vi "数据时间对齐.vi"(9 "待对齐时间":T1 {"单位" items=["ug/L", "mg/L", "ppm", "mg/m3", "cm", "ppb", "ug/m3", "%", "nmol/mol", "umol/mol", "MPN/L", "MPN/100ml", "ng/m3", "NTU", "无量纲", "ms/cm", "us/cm", "℃", "mV", "万个/L"]}, 10 "对齐参考时间":T1 {"单位" items=["ug/L", "mg/L", "ppm", "mg/m3", "cm", "ppb", "ug/m3", "%", "nmol/mol", "umol/mol", "MPN/L", "MPN/100ml", "ng/m3", "NTU", "无量纲", "ms/cm", "us/cm", "℃", "mV", "万个/L"]}, 11 "已对齐时间输入":T1 {"单位" items=["ug/L", "mg/L", "ppm", "mg/m3", "cm", "ppb", "ug/m3", "%", "nmol/mol", "umol/mol", "MPN/L", "MPN/100ml", "ng/m3", "NTU", "无量纲", "ms/cm", "us/cm", "℃", "mV", "万个/L"]}) -> (3 "已对齐时间输出":T1 {"单位" items=["ug/L", "mg/L", "ppm", "mg/m3", "cm", "ppb", "ug/m3", "%", "nmol/mol", "umol/mol", "MPN/L", "MPN/100ml", "ng/m3", "NTU", "无量纲", "ms/cm", "us/cm", "℃", "mV", "万个/L"]})   [LabVIEW 2022 SP3, in "斯坦道总磷总氮.lvlib"]
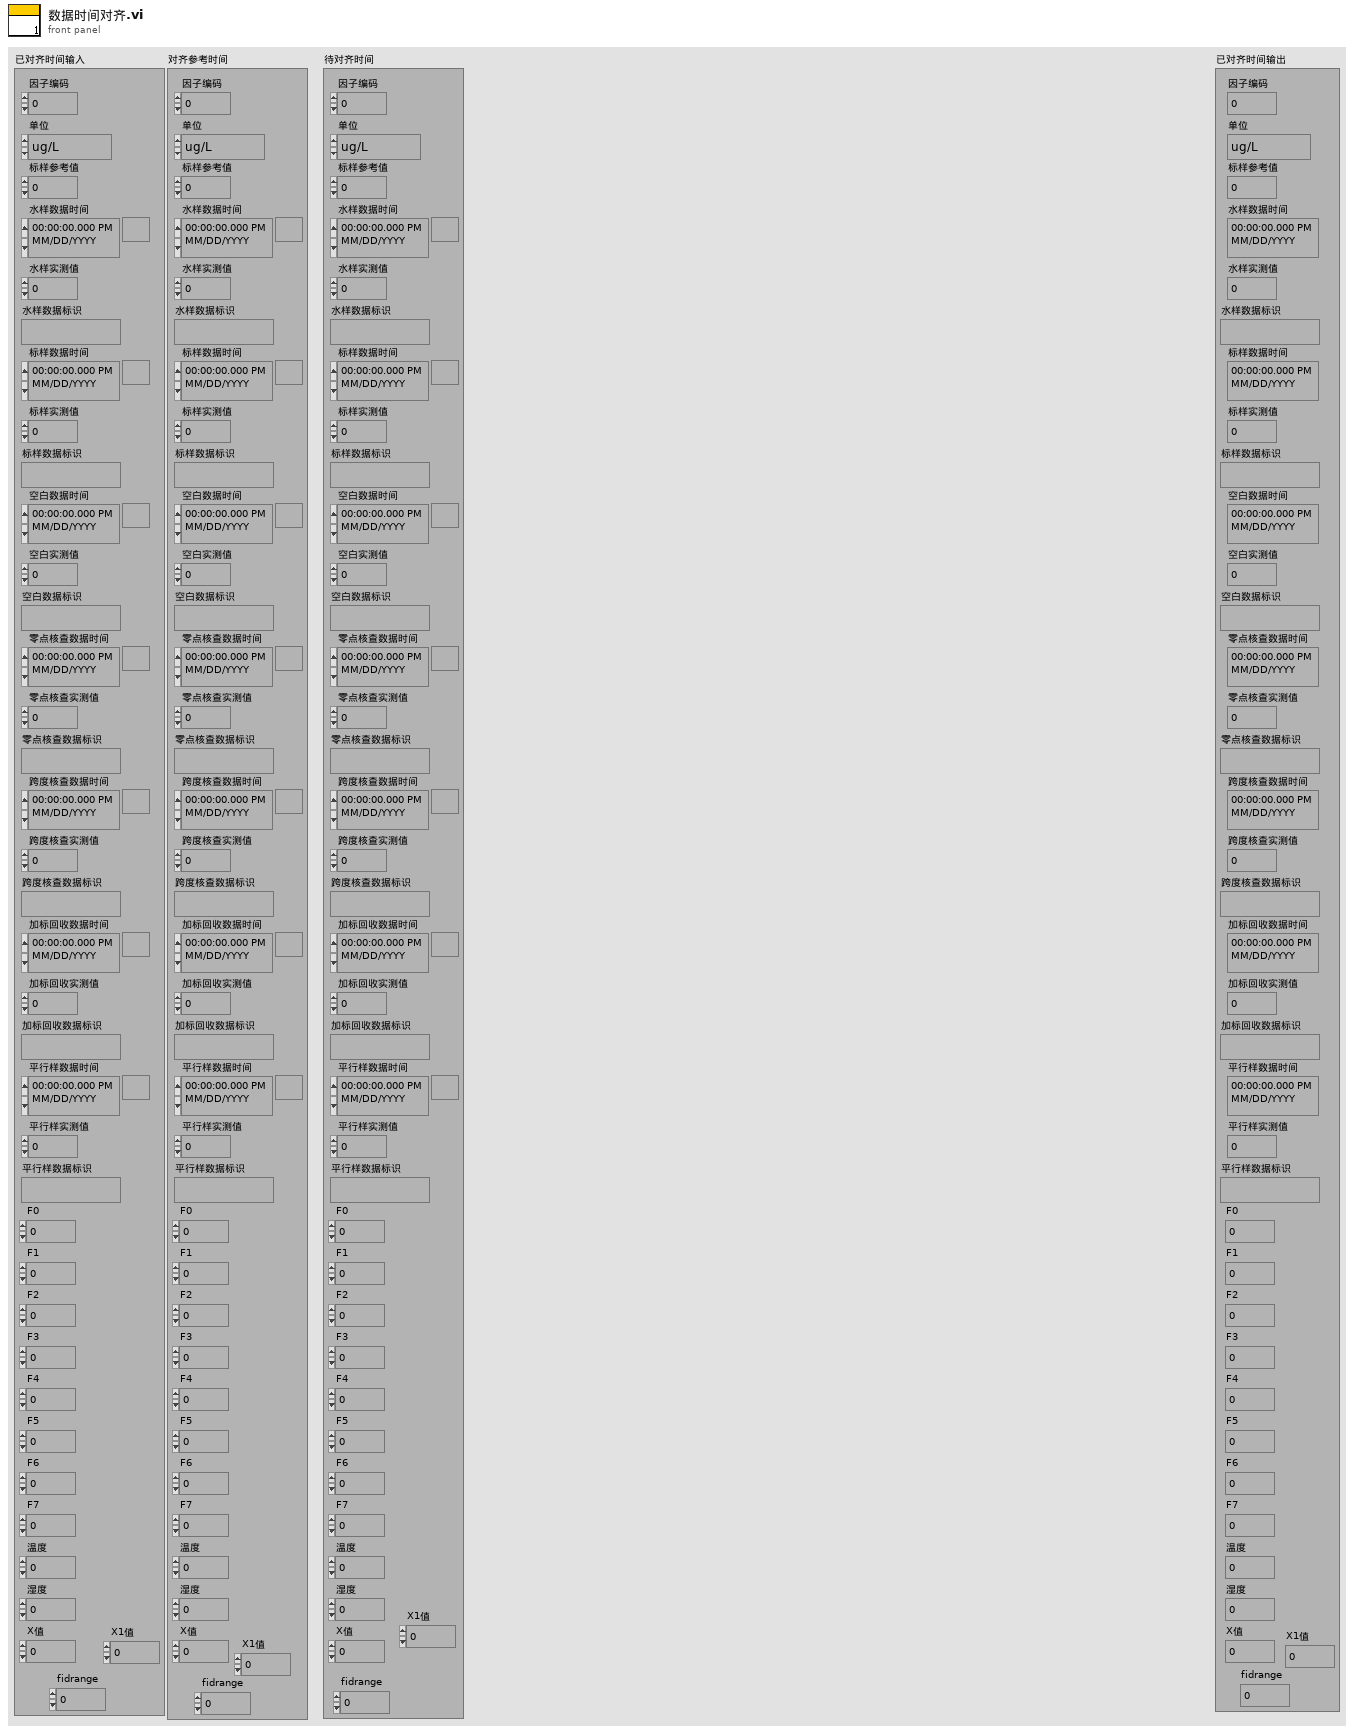
[diagram p1: front panel]
types:
  T1 = cluster{"因子编码":u32, "单位":u16, "标样参考值":sgl, "水样数据时间":timestamp, "水样实测值":sgl, "水样数据标识":string, "标样数据时间":timestamp, "标样实测值":sgl, "标样数据标识":string, "空白数据时间":timestamp, "空白实测值":sgl, "空白数据标识":string, "零点核查数据时间":timestamp, "零点核查实测值":sgl, "零点核查数据标识":string, "跨度核查数据时间":timestamp, "跨度核查实测值":sgl, "跨度核查数据标识":string, "加标回收数据时间":timestamp, "加标回收实测值":sgl, "加标回收数据标识":string, "平行样数据时间":timestamp, "平行样实测值":sgl, "平行样数据标识":string, "F0":sgl, "F1":sgl, "F2":sgl, "F3":sgl, "F4":sgl, "F5":sgl, "F6":sgl, "F7":sgl, "温度":sgl, "湿度":sgl, "X值":sgl, "fidrange":u16, "X1值":sgl}
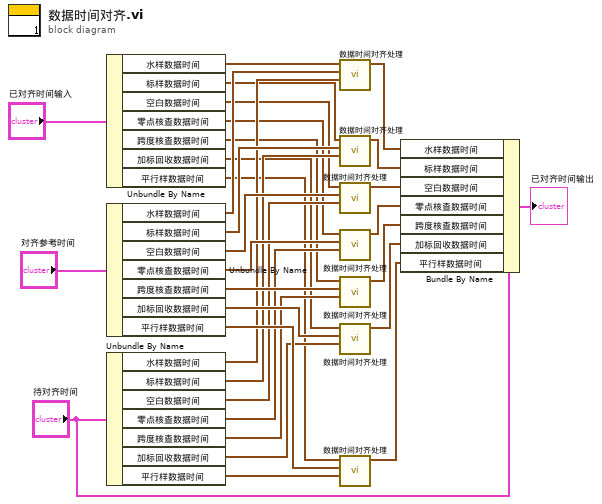
[diagram p0: block diagram]
diagram:
  n1 = Unbundle By Name("已对齐时间输入") -> ("水样数据时间"=w15:timestamp, "标样数据时间"=w13:timestamp, "空白数据时间"=w11:timestamp, "零点核查数据时间"=w9:timestamp, "跨度核查数据时间"=w7:timestamp, "加标回收数据时间"=w5:timestamp, "平行样数据时间"=w3:timestamp)
  n2 = Unbundle By Name("对齐参考时间") -> ("水样数据时间"=w24:timestamp, "标样数据时间"=w25:timestamp, "空白数据时间"=w26:timestamp, "零点核查数据时间"=w27:timestamp, "跨度核查数据时间"=w28:timestamp, "加标回收数据时间"=w29:timestamp, "平行样数据时间"=w30:timestamp)
  n3 = Unbundle By Name("待对齐时间") -> ("水样数据时间"=w17:timestamp, "标样数据时间"=w18:timestamp, "空白数据时间"=w19:timestamp, "零点核查数据时间"=w20:timestamp, "跨度核查数据时间"=w21:timestamp, "加标回收数据时间"=w22:timestamp, "平行样数据时间"=w23:timestamp)
  n4 = call "数据时间对齐处理.vi"("待对齐时间"=w17, "对齐参考时间"=w24, "已对齐时间输入"=w15) -> ("已对齐时间输出"=w14:timestamp)  [unwired: 8 in]
  n5 = call "数据时间对齐处理.vi"("待对齐时间"=w18, "对齐参考时间"=w25, "已对齐时间输入"=w13) -> ("已对齐时间输出"=w12:timestamp)  [unwired: 8 in]
  n6 = call "数据时间对齐处理.vi"("待对齐时间"=w19, "对齐参考时间"=w26, "已对齐时间输入"=w11) -> ("已对齐时间输出"=w10:timestamp)  [unwired: 8 in]
  n7 = call "数据时间对齐处理.vi"("待对齐时间"=w20, "对齐参考时间"=w27, "已对齐时间输入"=w9) -> ("已对齐时间输出"=w8:timestamp)  [unwired: 8 in]
  n8 = call "数据时间对齐处理.vi"("待对齐时间"=w21, "对齐参考时间"=w28, "已对齐时间输入"=w7) -> ("已对齐时间输出"=w6:timestamp)  [unwired: 8 in]
  n9 = call "数据时间对齐处理.vi"("待对齐时间"=w22, "对齐参考时间"=w29, "已对齐时间输入"=w5) -> ("已对齐时间输出"=w4:timestamp)  [unwired: 8 in]
  n10 = call "数据时间对齐处理.vi"("待对齐时间"=w23, "对齐参考时间"=w30, "已对齐时间输入"=w3) -> ("已对齐时间输出"=w2:timestamp)  [unwired: 8 in]
  n11 = Bundle By Name(cluster="待对齐时间", "水样数据时间"=w14, "标样数据时间"=w12, "空白数据时间"=w10, "零点核查数据时间"=w8, "跨度核查数据时间"=w6, "加标回收数据时间"=w4, "平行样数据时间"=w2) -> (→"已对齐时间输出":T1)
